vi "GetErrors3.vi"(0 "XRef":T6, 1 "Generate Strings?":T1, 2 "State In":T5) -> (14 "Errors":T2, 15 "Errors Present?":T1)   [LabVIEW 2012, in "CThread.lvlib" / "CThread VI Terminal Node.xnode"]
doc: "This ability VI is used to tell LabVIEW about errors involving your XNode instance. The Errors array is a cluster of errors that will show up as block diagram errors in LabVIEW's error window. The cluster is made up of the errors in the list, the long descriptions of the errors that show up in LabVIEW's error window's details box, and a help file and topic within that file that links this error to the specified help file via the Help button. The help file is the name of the file (*.chm), not the full path and needs to be part of LabVIEW. You only need to populate the array when Generate Strings? is true. You always need to correctly set the Errors Present? indicator. If you are generating strings, then Errors Present? should be true if and only if Errors is not empty. If errors are present, the VI containing the XNode will be broken.\n \n Remeber to localize your errors.\n\nDefault behavior: Generate generic error messages if the code you script is invalid, or a required terminal is unwired.\n\nThis ability does not provide UI and OS messages are not handled."
uses:
  CThread VI Terminal Node.xnode
  <vilib>/XNodeSupport/XNodeXNodeRef.ctl
  <vilib>/XNodeSupport/XNodeBool.ctl
  State.ctl
  <vilib>/XNodeSupport/XNodeError3Array.ctl
  <vilib>/XNodeSupport/XNodeError3.ctl
  <vilib>/XNodeSupport/XNodeString.ctl
  <vilib>/XNodeSupport/NI_XNodeSupport.lvlib
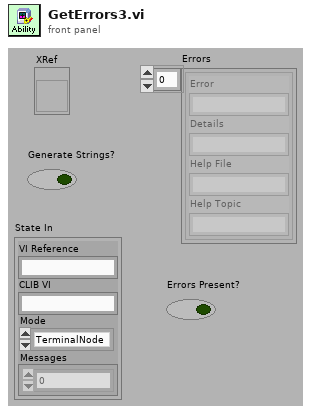
[diagram p1: front panel]
types:
  T1 = typedef "NI_XNodeSupport.lvlib/XNodeBool.ctl" = bool
  T2 = typedef "NI_XNodeSupport.lvlib/XNodeError3Array.ctl" = T3[]
  T3 = typedef "NI_XNodeSupport.lvlib/XNodeError3.ctl" = cluster{"Error":T4, "Details":T4, "Help File":T4, "Help Topic":T4}
  T4 = typedef "NI_XNodeSupport.lvlib/XNodeString.ctl" = string
  T5 = typedef "CThread.lvlib/CThread VI Terminal Node.xnode/State.ctl" = cluster{"VI Reference":string, "CLIB VI":string, "Mode":enum16{"TerminalNode", "AdaptorNode"}, "Messages":u8[]}
  T6 = typedef "NI_XNodeSupport.lvlib/XNodeXNodeRef.ctl" = refnum<vi>
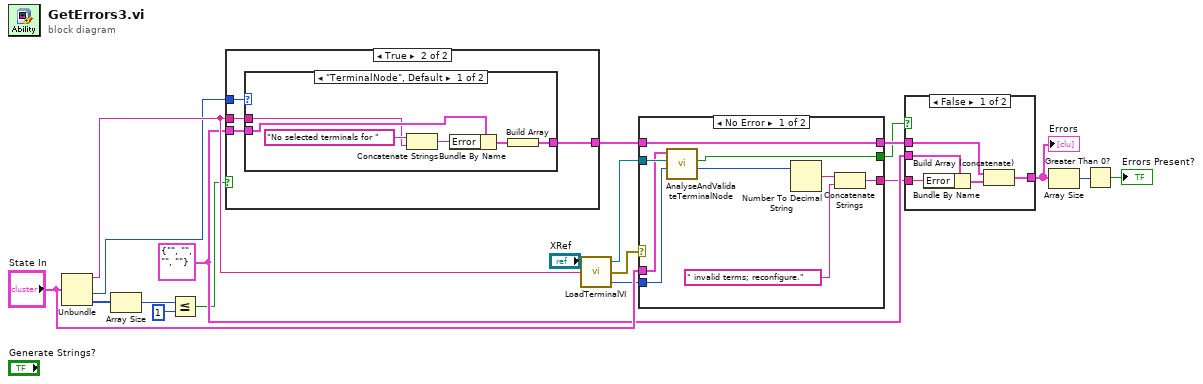
[diagram p0: block diagram]
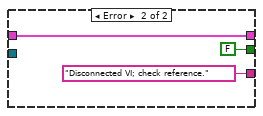
[diagram p3: hidden frame]
diagram:
  w9 = T3 {"Error"="", "Details"="", "Help File"="", "Help Topic"=""} ("Error 3")
  n1 = Unbundle("State In") -> ("VI Reference"=w16:string, "Mode"=w2:enum16{"TerminalNode", "AdaptorNode"}, "Messages"=w19:u8[])  [unwired: 1 out]
  n2 = Array Size(array=w19) -> (size(s)=w4:i32)
  n3 = Less Or Equal?(x=w4, y=1) -> (x <= y?=w5:bool)
  n4 = case shown="True" w5 {
    tunnel: w9 -> [_ w23]
    tunnel: [_ w22] -> w7
    tunnel: w16 -> [_ w21]
    tunnel: w2 -> [_ w20]
    frame False {
    }
    frame True {
      n5 = case shown="\"TerminalNode\", Default" w20 {
        tunnel: w23 -> [w27 _]
        tunnel: [w25 _] -> w22
        tunnel: w21 -> [w24 _]
        frame "TerminalNode", Default {
          n6 = Concatenate Strings("No selected terminals for " ("string"), w24) -> (w28:string)
          n7 = Bundle By Name(cluster=w27, "Error"=w28) -> (w26:T3)
          n8 = Build Array(w26) -> (w25:T3[])
        }
        frame "AdaptorNode" {
        }
      }
    }
  }
  n9 = call "LoadTerminalVI.vi"("VI Reference"=w16, "XRef"="XRef") -> ("Clone Number"=w1:i16, "error out"=w13:errorcluster, "vi reference"=w14:refnum<vi>)  [unwired: 1 in]
  n10 = case shown="No Error" w13 {
    tunnel: w14 -> [w38 _]
    tunnel: "State In" -> [w37 _]
    tunnel: w7 -> [w36 w41]
    tunnel: [w36 w41] -> w11
    tunnel: [w35 FALSE ("Valid")] -> w10
    tunnel: [w34 "Disconnected VI; check reference."] -> w8
    tunnel: w1 -> [w30 _]
    frame No Error {
      n11 = call "AnalyseAndValidateTerminalNode.vi"("CloneID"=w30, "Comparison VI"=w38, "State"=w37) -> ("Invalid Terms"=w33:u8, "Valid"=w35:bool)  [unwired: 5 in, 2 out]
      n12 = Number To Decimal String(number=w33) -> (decimal integer string=w32:string)  [unwired: 1 in]
      n13 = Concatenate Strings(w32, " invalid terms; reconfigure." ("string")) -> (w34:string)
    }
    frame Error {
    }
  }
  n14 = case shown="False" w10 {
    tunnel: w11 -> [w45 w47]
    tunnel: w9 -> [w44 _]
    tunnel: w8 -> [w43 _]
    tunnel: [w42 w47] -> w6
    frame False {
      n15 = Bundle By Name(cluster=w44, "Error"=w43) -> (w46:T3)
      n16 = Build Array (concatenate)(w45, w46) -> (w42:T3[])
    }
    frame True {
    }
  }
  "Errors" <- w6
  n17 = Array Size(array=w6) -> (size(s)=w18:i32)
  n18 = Greater Than 0?(x=w18) -> (x > 0?=→"Errors Present?":bool)
